vi "Remove Connection.vi"(8 "error in (no error)":errorcluster, 9 "channel 2":string, 10 "channel 1":string, 11 "SLSC Switch in":refnum<class "SLSC Switch.lvclass">) -> (0 "error out":errorcluster, 3 "SLSC Switch out":refnum<class "SLSC Switch.lvclass">)   [LabVIEW 2015, in "SLSC Switch.lvlib" / "SLSC Switch.lvclass"]
uses:
  SLSC Switch.lvclass
  Controls/Connection.ctl
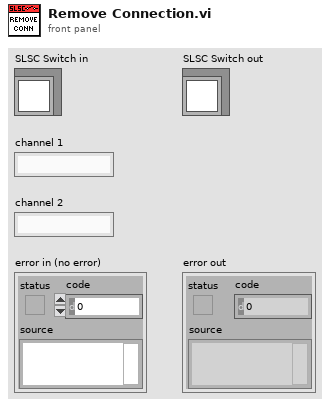
[diagram p1: front panel]
types:
  T1 = typedef "SLSC Switch.lvlib/SLSC Switch.lvclass/Connection.ctl" = cluster{"channel 1":string, "channel 2":string}
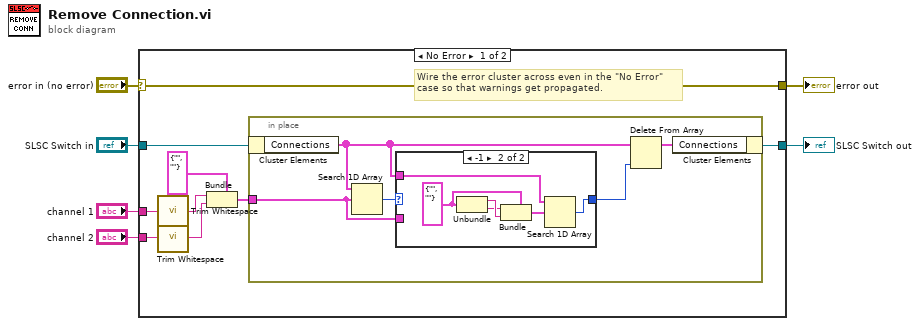
[diagram p0: block diagram]
diagram:
  n1 = case shown="No Error" "error in (no error)" {
    selector: "error in (no error)" -> [w15 w29]
    tunnel: [w15 w29] -> w5
    tunnel: [w13 w28] -> w3
    tunnel: "SLSC Switch in" -> [w14 w28]
    tunnel: "channel 1" -> [w10 _]
    tunnel: "channel 2" -> [w9 _]
    frame No Error {
      # "Wire the error cluster across even in the \"No Error\"\ncase so that warnings get propagated."
      n2 = call <vilib>:"Trim Whitespace.vi"("string"=w10) -> ("trimmed string"=w8:string)  [unwired: 1 in]
      n3 = call <vilib>:"Trim Whitespace.vi"("string"=w9) -> ("trimmed string"=w7:string)  [unwired: 1 in]
      n4 = Bundle(cluster=T1 {"channel 1"="", "channel 2"=""} ("connections"), "channel 1"=w8, "channel 2"=w7) -> (w11:T1)
      n5 = in-place {
        in-place-border: w11 -> [w19]
        n6 = in-place-cluster #1(w14) -> ("Connections"=w18:T1[])
        n7 = Search 1D Array(1D array=w18, element=w19) -> (index of element=w20:i32)  [unwired: 1 in]
        n8 = case shown="-1" w20 {
          selector: w20 -> [w21 _]
          tunnel: w19 -> [_ _]
          tunnel: w18 -> [_ w23]
          tunnel: [w21 w22] -> w17
          frame 0, Default {
          }
          frame -1 {
            w27 = T1 {"channel 1"="", "channel 2"=""} ("connections")
            n9 = Unbundle(w27) -> ("channel 1"=w26:string, "channel 2"=w25:string)
            n10 = Bundle(cluster=w27, "channel 1"=w25, "channel 2"=w26) -> (w24:T1)
            n11 = Search 1D Array(1D array=w23, element=w24) -> (index of element=w22:i32)  [unwired: 1 in]
          }
        }
        n12 = Delete From Array(array=w18, index=w17) -> (array with subset deleted=w16:T1[])  [unwired: 1 in, 1 out]
        n13 = in-place-cluster #1("Connections"=w16) -> (w13:refnum<class "SLSC Switch.lvclass">)
      }
    }
    frame Error {
    }
  }
  "error out" <- w5
  "SLSC Switch out" <- w3
